vi "Run Output Actor.vi"(8 "error in (no error)":errorcluster, 11 "output_actor.lvclass":refnum<class "Output Actor.lvclass">) -> (0 "error out":errorcluster, 3 "Output Actor Interface":refnum<class "Output Actor Interface.lvclass">)   [LabVIEW 2015, in "Output Actor Interface.lvclass"]
uses:
  Output Actor Interface.lvclass
  Output Actor.lvclass
  Output Actor.lvclass/Output Actor.ctl
  Output Actor Interface.lvclass/Output Actor Interface.ctl
  <vilib>/ActorFramework/Actor/Actor.lvclass
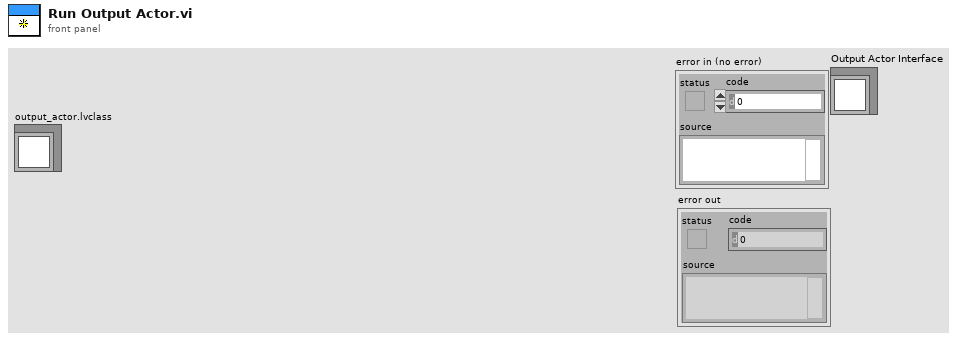
[diagram p1: front panel]
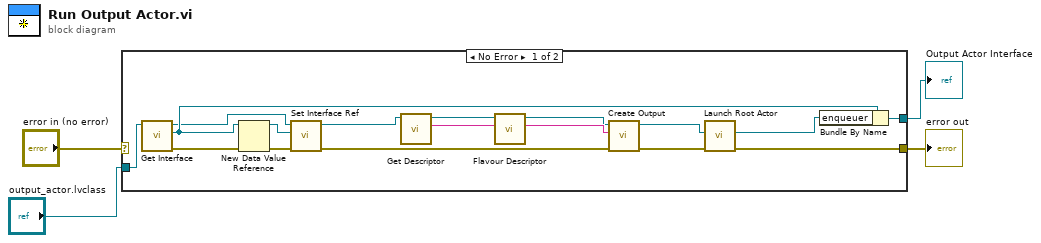
[diagram p0: block diagram]
diagram:
  n1 = case shown="No Error" "error in (no error)" {
    selector: "error in (no error)" -> [_ w22]
    tunnel: [w19 w22] -> w3
    tunnel: "output_actor.lvclass" -> [w9 _]
    tunnel: [w13 _] -> w1
    frame No Error {
      n2 = call-dynamic "Get Interface.vi"("Output Actor in"=w9) -> ("error out"=w11:errorcluster, "Output Actor Interface"=w12:refnum<class "Output Actor Interface.lvclass">, "Output Actor out"=w10:refnum<class "Output Actor.lvclass">)  [unwired: 8 in]
      n3 = New Data Value Reference(data value=w12, error in=w11) -> (data value reference=w21:refnum<data-value>, error out=w20:errorcluster)
      n4 = call "Set Interface Ref.vi"("error in (no error)"=w20, "interface ref"=w21, "output_actor in"=w10) -> ("error out"=w7:errorcluster, "output_actor out"=w8:refnum<class "Output Actor.lvclass">)  [unwired: 7 in]
      n5 = call-dynamic "Get Descriptor.vi"("output_actor in"=w8) -> ("Descriptor"=w17:string, "output_actor out"=w18:refnum<class "Output Actor.lvclass">)  [unwired: 9 in]
      n6 = call-dynamic "Flavour Descriptor.vi"("Descriptor"=w17, "output_actor in"=w18) -> ("Flavoured Descriptor"=w16:string, "output_actor out"=w15:refnum<class "Output Actor.lvclass">)  [unwired: 8 in]
      n7 = call "Create Output.vi"("error in (no error)"=w7, "Descriptor"=w16, "output_actor in"=w15) -> ("error out"=w5:errorcluster, "output_actor out"=w6:refnum<class "Output Actor.lvclass">)  [unwired: 7 in]
      n8 = call <vilib>:"Launch Root Actor.vi"("error in (no error)"=w5, "Actor"=w6) -> ("error out"=w19:errorcluster, "Actor's Enqueuer"=w14:refnum<class "Message Enqueuer.lvclass">)  [unwired: 8 in]
      n9 = Bundle By Name(cluster=w12, "enqueuer"=w14) -> (w13:refnum<class "Output Actor Interface.lvclass">)
    }
    frame Error {
    }
  }
  "error out" <- w3
  "Output Actor Interface" <- w1
